vi "svc_Sort Array (DBL).vi"(9 "sort order":u16(ring)=1 items=["Ascending", "Descending"], 11 "array":dbl[](array[numeric])) -> (2 "sort indices":i32[](array[numeric]), 3 "sorted array":dbl[](array[numeric]))   [LabVIEW 2017]
doc: "Sorts an array of peaks according to the <B>sort by</B> and <B>sort order</B> parameters. Use this VI to sort peaks that the SVFA Spectrum Peak Search, SVT Spurious Free Dynamic Range, and SVT THD and Harmonic Components VIs return. Wire data to the<B> peaks in</B> input to determine the polymorphic instance to use or manually select the instance."
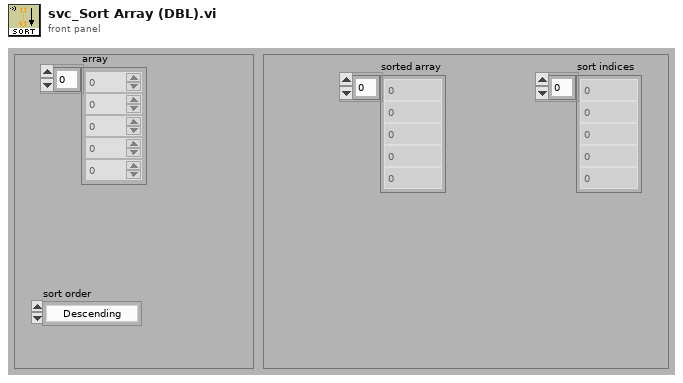
[diagram p1: front panel]
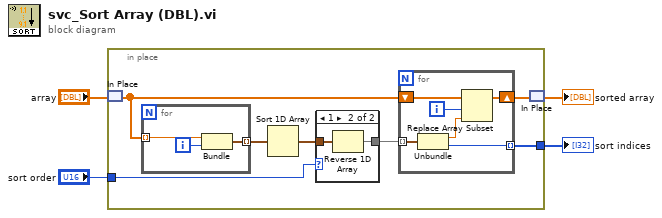
[diagram p0: block diagram]
diagram:
  n1 = in-place {
    in-place-border: "sort order" -> [w11]
    in-place-border: [w9] -> w3
    n2 = in-place-match #1("array") -> (w6:dbl[])
    n3 = for {
      tunnel: [w20] -> w8 mode=indexing
      tunnel: w6 -> [w18] mode=indexing
      i -> [w19]
      n4 = Bundle("X"=w18, w19) -> (w20:cluster{"X":dbl, i32})  [unwired: 1 in]
    }
    n5 = Sort 1D Array(array=w8) -> (sorted array=w7:cluster{"X":dbl, i32}[])
    n6 = case shown="1" w11 {
      tunnel: [w21 w23] -> w10
      tunnel: w7 -> [w21 w22]
      frame 0, Default {
      }
      frame 1 {
        n7 = Reverse 1D Array(array=w22) -> (reversed array=w23:cluster{"X":dbl, i32}[])
      }
    }
    n8 = for {
      tunnel: w10 -> [w17] mode=indexing
      tunnel: [w16] -> w9 mode=indexing
      shift-right: [w15] -> w5
      shift-left: w6 -> [w14]
      i -> [w13]
      n9 = Unbundle(w17) -> ("X"=w12:dbl, w16:i32)
      n10 = Replace Array Subset(array=w14, new element=w12, index=w13) -> (w15:dbl[])
    }
    n11 = in-place-match #1(w5) -> (→"sorted array":dbl[])
  }
  "sort indices" <- w3
